vi "Tool tulle data.vi"(1 "Action(GET)":enum16{"GET", "SET"}(ring), 7 "Tool Data in":T5 {"DH.Modem"."Pin.mA" scale=0.0..200.0; "DH.Modem"."Pin.V" scale=0.0..36.0; "DH.PSU"."Temp" scale=0.0..200.0; "DH.PSU"."24v.A" scale=0.0..4.0; "DH.PSU"."24v.V" scale=0.0..36.0; "DH.PSU"."Pin.mA" scale=0.0..1000.0; "DH.PSU"."Pin.V" scale=0.0..1000.0; "DH.Controller"."Temp" scale=0.0..200.0; "DH.Controller"."Ain.4 v" scale=0.0..10.0; "DH.Controller"."Ain.3 v" scale=0.0..10.0; "DH.Controller"."Ain.2 v" scale=0.0..10.0; "DH.Controller"."Ain.1 v" scale=0.0..10.0; "DH.Controller"."Acc.Z g" scale=-6.0..6.0; "DH.Controller"."Acc.Y g" scale=-6.0..6.0; "DH.Controller"."Acc.X g" scale=-6.0..6.0; "DH.Controller"."Pin.A" scale=0.0..4.0; "DH.Controller"."Pin.V" scale=0.0..36.0; "DH.Solonoid driver"."L.cur 6" scale=0.0..2.0; "DH.Solonoid driver"."L.cur 5" scale=0.0..2.0; "DH.Solonoid driver"."L.cur 4" scale=0.0..2.0; "DH.Solonoid driver"."L.cur 3" scale=0.0..2.0; "DH.Solonoid driver"."L.cur 2" scale=0.0..2.0; "DH.Solonoid driver"."L.cur 1" scale=0.0..2.0; "DH.Solonoid driver"."Stroke mm" scale=0.0..500.0; "DH.Solonoid driver"."Temp" scale=0.0..200.0}, 11 "error in (no error)":errorcluster) -> (8 "Tool Data out":T5 {"DH.Modem"."Pin.mA" scale=0.0..200.0; "DH.Modem"."Pin.V" scale=0.0..36.0; "DH.PSU"."Temp" scale=0.0..200.0; "DH.PSU"."24v.A" scale=0.0..4.0; "DH.PSU"."24v.V" scale=0.0..36.0; "DH.PSU"."Pin.mA" scale=0.0..1000.0; "DH.PSU"."Pin.V" scale=0.0..1000.0; "DH.Controller"."Temp" scale=0.0..200.0; "DH.Controller"."Ain.4 v" scale=0.0..10.0; "DH.Controller"."Ain.3 v" scale=0.0..10.0; "DH.Controller"."Ain.2 v" scale=0.0..10.0; "DH.Controller"."Ain.1 v" scale=0.0..10.0; "DH.Controller"."Acc.Z g" scale=-6.0..6.0; "DH.Controller"."Acc.Y g" scale=-6.0..6.0; "DH.Controller"."Acc.X g" scale=-6.0..6.0; "DH.Controller"."Pin.A" scale=0.0..4.0; "DH.Controller"."Pin.V" scale=0.0..36.0; "DH.Solonoid driver"."L.cur 6" scale=0.0..2.0; "DH.Solonoid driver"."L.cur 5" scale=0.0..2.0; "DH.Solonoid driver"."L.cur 4" scale=0.0..2.0; "DH.Solonoid driver"."L.cur 3" scale=0.0..2.0; "DH.Solonoid driver"."L.cur 2" scale=0.0..2.0; "DH.Solonoid driver"."L.cur 1" scale=0.0..2.0; "DH.Solonoid driver"."Stroke mm" scale=0.0..500.0; "DH.Solonoid driver"."Temp" scale=0.0..200.0}, 15 "error out":errorcluster)   [LabVIEW 2011]
uses:
  Tool/Stroker/def/Tool Stroker Modem ana.ctl
  Tool/Stroker/def/Tool Stroker PSU ana.ctl
  Tool/Stroker/def/Tool Stroker Controller ana.ctl
  Tool/Stroker/def/Tool Stroker Solonoid ana.ctl
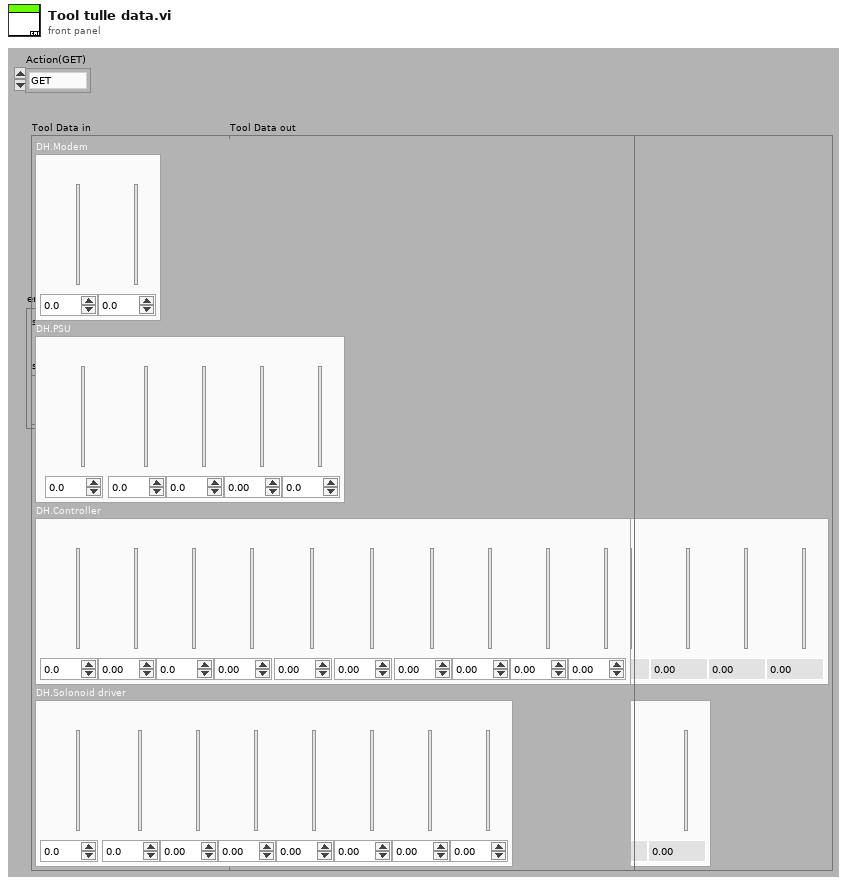
[diagram p1: front panel]
types:
  T1 = typedef "Tool Stroker Modem ana.ctl" = cluster{"Pin.V":dbl, "Pin.mA":dbl}
  T2 = typedef "Tool Stroker PSU ana.ctl" = cluster{"Pin.V":dbl, "Pin.mA":dbl, "24v.V":dbl, "24v.A":dbl, "Temp":dbl}
  T3 = typedef "Tool Stroker Controller ana.ctl" = cluster{"Pin.V":dbl, "Pin.A":dbl, "Temp":dbl, "Acc.X g":dbl, "Acc.Y g":dbl, "Acc.Z g":dbl, "Ain.1 v":dbl, "Ain.2 v":dbl, "Ain.3 v":dbl, "Ain.4 v":dbl}
  T4 = typedef "Tool Stroker Solonoid ana.ctl" = cluster{"Stroke mm":dbl, "Temp":dbl, "L.cur 1":dbl, "L.cur 2":dbl, "L.cur 3":dbl, "L.cur 4":dbl, "L.cur 5":dbl, "L.cur 6":dbl}
  T5 = cluster{"DH.Modem":T1, "DH.PSU":T2, "DH.Controller":T3, "DH.Solonoid driver":T4}
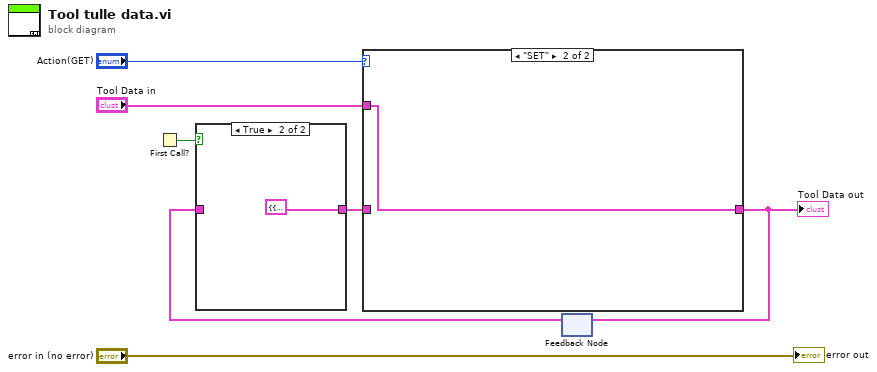
[diagram p0: block diagram]
diagram:
  n1 = First Call?() -> (First Call?: T/F=w4:bool)
  n2 = feedback #1() -> (w5:T5)  [unwired: 1 in]
  n3 = case shown="True" w4 {
    tunnel: w5 -> [w8 _]
    tunnel: [w8 T5 {"DH.Modem"={"Pin.V"=0.0, "Pin.mA"=0.0}, "DH.PSU"={"Pin.V"=0.0, "Pin.mA"=0.0, "24v.V"=0.0, "24v.A"=0.0, "Temp"=0.0}, "DH.Controller"={"Pin.V"=0.0, "Pin.A"=0.0, "Temp"=0.0, "Acc.X g"=0.0, "Acc.Y g"=0.0, "Acc.Z g"=0.0, "Ain.1 v"=0.0, "Ain.2 v"=0.0, "Ain.3 v"=0.0, "Ain.4 v"=0.0}, "DH.Solonoid driver"={"Stroke mm"=0.0, "Temp"=0.0, "L.cur 1"=0.0, "L.cur 2"=0.0, "L.cur 3"=0.0, "L.cur 4"=0.0, "L.cur 5"=0.0, "L.cur 6"=0.0}} ("Tool Data")] -> w2
    frame False {
    }
    frame True {
    }
  }
  n4 = case shown="\"SET\"" "Action(GET)" {
    tunnel: [w10 w11] -> w3
    tunnel: w2 -> [w10 _]
    tunnel: "Tool Data in" -> [_ w11]
    frame "GET", Default {
    }
    frame "SET" {
    }
  }
  "Tool Data out" <- w3
  n5 = feedback-in #1(w3) -> ()
  "error out" <- "error in (no error)"
